vi "q5 threshold operation.vi"() -> ()   [LabVIEW 2018]
uses:
  <vilib>/vision/NI_Vision_Development_Module.lvlib
panel:
  in  "Range":cluster{"Lower value":sgl, "Upper value":sgl}={"Lower value"=128.0, "Upper value"=255.0} {"Upper value" format="%.2f"; "Lower value" format="%.2f"}
  out "Image 2":T1(plugin-control)
  in  "Replace Value":sgl=1.0 format="%.2f"
  in  "Keep/Replace Value (Replace)":bool=TRUE
  in  "Use File Path Image Type":bool=TRUE
  out "Image":T1(plugin-control)
  in  "File Path":path
  in  "Image Type":T2 items=["Grayscale (U8)", "Grayscale (I16)", "Grayscale (SGL)", "Complex (CSG)", "RGB (U32)", "HSL (U32)", "RGB (U64)", "Grayscale (U16)"]
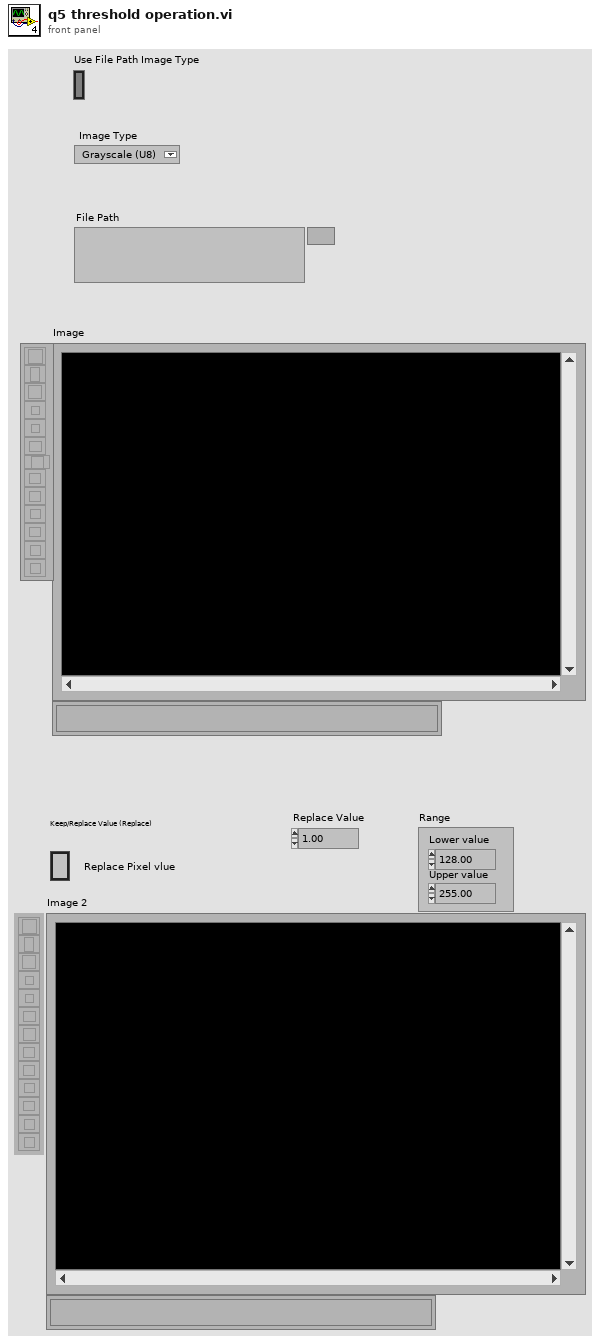
[diagram p1: front panel]
types:
  T1 = typedef "IMAQ Image.ctl" = refnum<image>
  T2 = typedef "Image Type" = u32
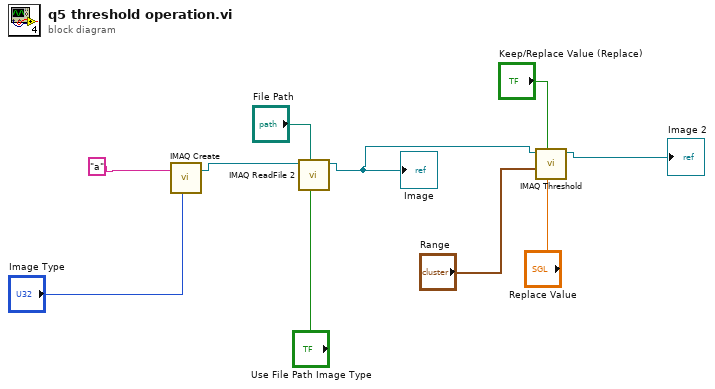
[diagram p0: block diagram]
diagram:
  n1 = call "IMAQ Create"("Image Name"="a", "Image Type"="Image Type") -> ("New Image"=w8:T1)  [unwired: 3 in, 1 out]
  n2 = call "IMAQ ReadFile 2"("Use File Path Image Type"="Use File Path Image Type", "File Path"="File Path", "Image"=w8) -> ("Image Out"=w5:T1)  [unwired: 4 in, 4 out]
  "Image" <- w5
  n3 = call "IMAQ Threshold"("Replace Value"="Replace Value", "Keep/Replace Value (Replace)"="Keep/Replace Value (Replace)", "Range"="Range", "Image Src"=w5) -> ("Image Dst Out"=→"Image 2":T1)  [unwired: 6 in, 1 out]
